vi "Resolve Link.vi"(5 "Username":string, 6 "Password":string, 7 "Address":string, 8 "Error In":errorcluster) -> (0 "Error Out":errorcluster)   [LabVIEW 2018, in "Tests.lvlib" / "SFTP.lvlib"]
uses:
  SFTP.lvlib
  src/Toolkit/API/SFTP File/API/Typedefs/Flags.ctl
  src/Toolkit/API/SFTP/Support/Resolve Real Link.vi
  <vilib>/addons/_JKI Toolkits/Caraya/classes/Test/Test.lvclass
  <vilib>/addons/_JKI Toolkits/Caraya/classes/Assert/Assert.lvclass
  src/Toolkit/API/SFTP/SFTP.lvclass
  src/Toolkit/API/SFTP File/SFTP File.lvclass
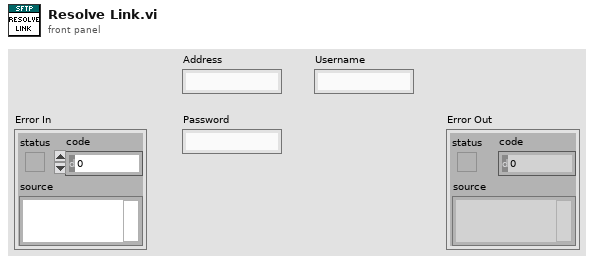
[diagram p1: front panel]
types:
  T1 = typedef "Toolkit.lvlib/SFTP File.lvclass/Flags.ctl" = cluster{"Read":bool, "Write":bool, "Append":bool, "Create":bool, "Truncate":bool, "Exclude":bool}
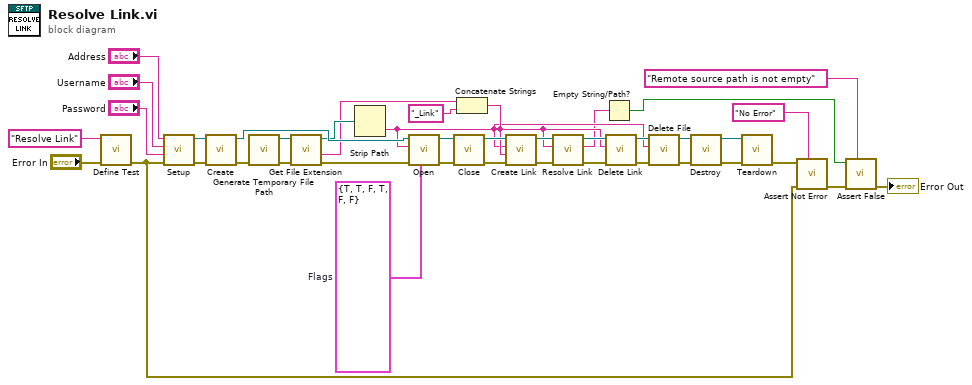
[diagram p0: block diagram]
diagram:
  w27 = T1 {"Read"=TRUE, "Write"=TRUE, "Append"=FALSE, "Create"=TRUE, "Truncate"=FALSE, "Exclude"=FALSE}  # Flags
  n1 = call <vilib>:"Define Test.vi"("error in (no error)"="Error In", "Label (VI Title)"="Resolve Link") -> ("error out"=w35:errorcluster)  [unwired: 9 in]
  n2 = call "Setup.vi"("Error In"=w35, "Password"="Password", "Username"="Username", "Address"="Address") -> ("Error Out"=w36:errorcluster, "Sesssion"=w31:refnum<class "Session.lvclass">)  [unwired: 6 in]
  n3 = call "Create.vi"("Error In"=w36, "Session"=w31) -> ("Error Out"=w24:errorcluster, "SFTP"=w23:refnum<class "SFTP.lvclass">)  [unwired: 8 in]
  n4 = call <vilib>:"Generate Temporary File Path.vi"("error in (no error)"=w24) -> ("error out"=w18:errorcluster, "Unique Temporary File Path"=w20:path)  [unwired: 9 in]
  n5 = call <vilib>:"Get File Extension.vi"("error in (no error)"=w18, "file"=w20) -> ("error out"=w17:errorcluster, "filename without extension"=w16:string, "dup file"=w19:path)  [unwired: 5 in, 2 out]
  n6 = Strip Path(path=w19) -> (name=w3:string)  [unwired: 1 out]
  n7 = call "Open.vi"("Flags"=w27, "Error In"=w17, "Remote Path"=w3, "SFTP"=w23) -> ("Error Out"=w25:errorcluster, "SFTP File"=w26:refnum<class "SFTP File.lvclass">)  [unwired: 6 in]
  n8 = call "Close.vi"("Error In"=w25, "SFTP File"=w26) -> ("Error Out"=w21:errorcluster, "SFTP"=w22:refnum<class "SFTP.lvclass">)  [unwired: 7 in, 1 out]
  n9 = Concatenate Strings(w16, "_Link" ("string")) -> (w4:string)
  n10 = call "Create Link.vi"("Error In"=w21, "Remote Link Path"=w4, "Remote Source Path"=w3, "SFTP In"=w22) -> ("Error Out"=w6:errorcluster, "SFTP Out"=w7:refnum<class "SFTP.lvclass">)  [unwired: 6 in]
  n11 = call-poly "Resolve Link.vi"("Error In"=w6, "Remote Link Path"=w4, "SFTP In"=w7) -> ("Error Out"=w5:errorcluster, "Remote Source Path"=w2:string, "SFTP Out"=w8:refnum<class "SFTP.lvclass">)  [unwired: 6 in]
  n12 = Empty String/Path?(string/path=w2) -> (empty?=w1:bool)
  n13 = call "Delete Link.vi"("Error In"=w5, "Remote Path"=w4, "SFTP In"=w8) -> ("Error Out"=w12:errorcluster, "SFTP Out"=w11:refnum<class "SFTP.lvclass">)  [unwired: 7 in]
  n14 = call "Delete File.vi"("Error In"=w12, "Remote Path"=w3, "SFTP In"=w11) -> ("Error Out"=w13:errorcluster, "SFTP Out"=w14:refnum<class "SFTP.lvclass">)  [unwired: 7 in]
  n15 = call "Destroy.vi"("Error In"=w13, "SFTP"=w14) -> ("Error Out"=w30:errorcluster, "Session"=w28:refnum<class "Session.lvclass">)  [unwired: 8 in]
  n16 = call "Teardown.vi"("Error In"=w30, "Session"=w28) -> ("Error Out"=w29:errorcluster)  [unwired: 9 in]
  n17 = call <vilib>:"Assert Not Error.vi"("Label"="No Error", "error in (no error)"=w35, "Not Error?"=w29) -> ("error out"=w37:errorcluster)  [unwired: 8 in]
  n18 = call <vilib>:"Assert False.vi"("Label"="Remote source path is not empty", "error in (no error)"=w37, "False?"=w1) -> ("error out"=→"Error Out":errorcluster)  [unwired: 8 in]
